vi "ColorImageTest.vi"() -> ()   [LabVIEW 2011]
uses:
  Microsoft.Kinect
  <vilib>/vision/NI_Vision_Development_Module.lvlib
panel:
  in  "ElevationAngle":i32 min=-27 max=27
  out "Iteration":i32
  in  "stop":bool
  in  "millisecondsWait":i32=1000
  out "error out":errorcluster
  out "Array":T1(array[cluster])
  out "Depth Frame":T2(plugin-control)
  out "BeamAngle":dbl
  out "SoundSourceAngle":dbl
  out "SoundSourceAngleConfidence":dbl
  out "Color Frame":T2(plugin-control)
  out "Color Pixel Data":u8[](array[numeric])
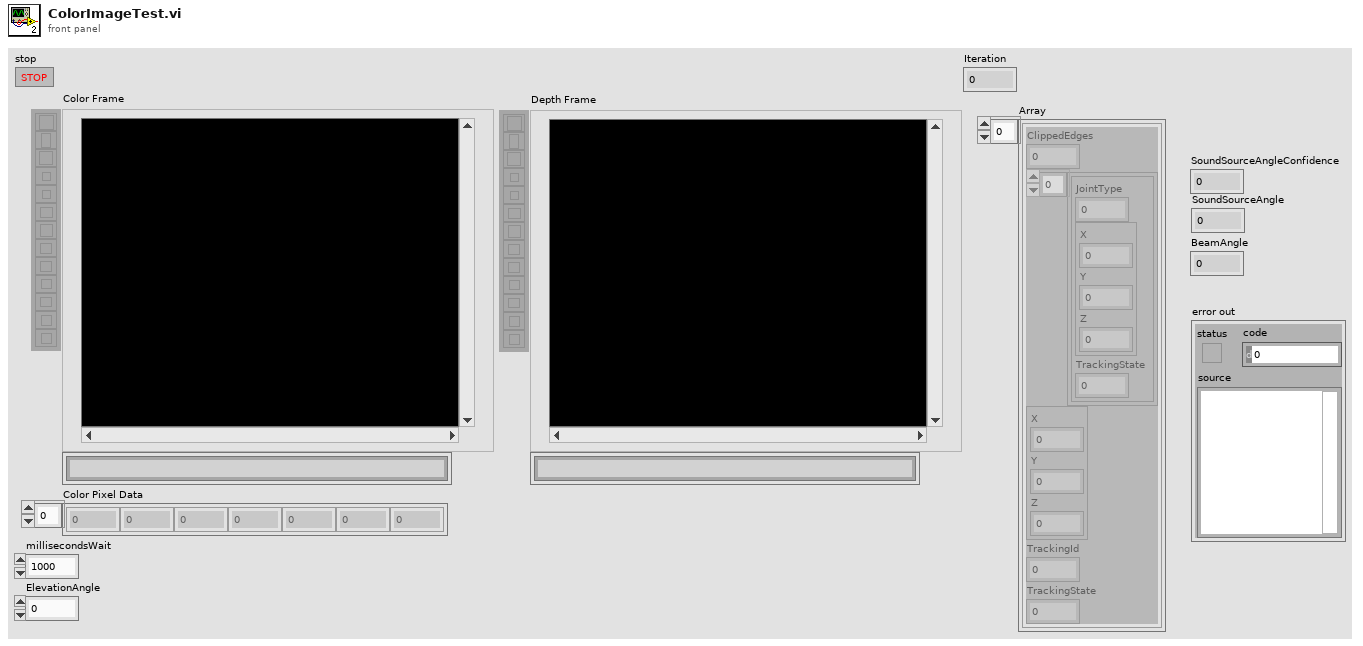
[diagram p1: front panel]
types:
  T1 = cluster{"ClippedEdges":i32, cluster{"JointType":i32, cluster{"X":sgl, "Y":sgl, "Z":sgl}, "TrackingState":i32}[], cluster{"X":sgl, "Y":sgl, "Z":sgl}, "TrackingId":i32, "TrackingState":i32}[]
  T2 = typedef "IMAQ Image.ctl" = refnum<image>
  T3 = typedef "Image Type" = u32
  T4 = cluster{"JointType":i32, cluster{"X":sgl, "Y":sgl, "Z":sgl}, "TrackingState":i32}
  T5 = cluster{"ClippedEdges":i32, cluster{"JointType":i32, cluster{"X":sgl, "Y":sgl, "Z":sgl}, "TrackingState":i32}[], cluster{"X":sgl, "Y":sgl, "Z":sgl}, "TrackingId":i32, "TrackingState":i32}
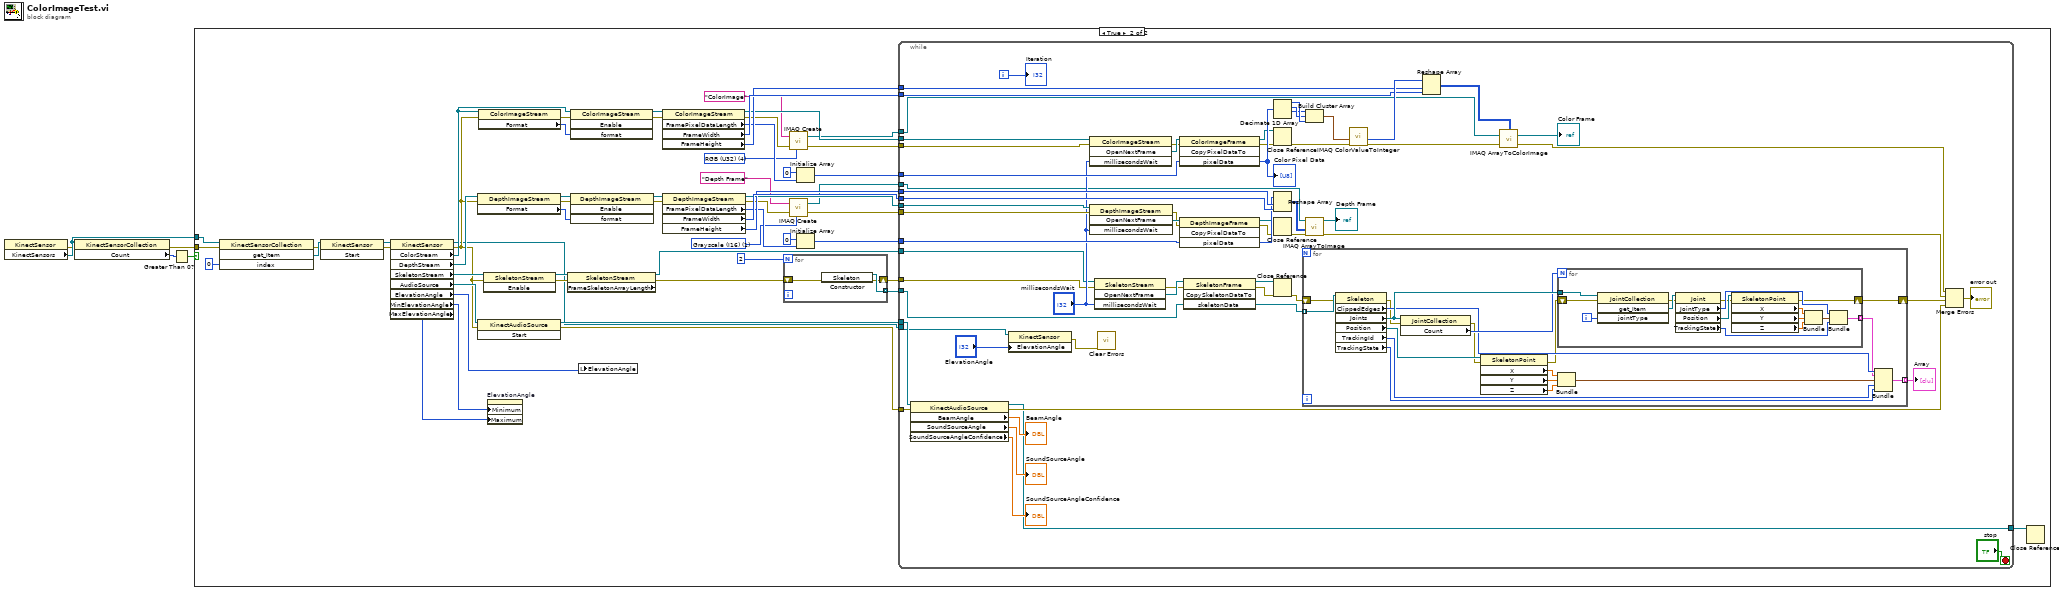
[diagram p0: block diagram]
diagram:
  n1 = property class="KinectSensor"() -> (error out=w2:errorcluster, "KinectSensors"=w5:refnum<k24>)  [unwired: 2 in, 1 out]
  n2 = property class="KinectSensorCollection"(reference=w5, error in=w2) -> (error out=w1:errorcluster, "Count"=w4:i32)  [unwired: 1 out]
  n3 = Greater Than 0?(x=w4) -> (x > 0?=w3:bool)
  n4 = case shown="True" w3 {
    tunnel: w5 -> [_ w62]
    tunnel: w1 -> [_ w48]
    frame False {
    }
    frame True {
      w19 = T3 4 items=["Grayscale (U8)", "Grayscale (I16)", "Grayscale (SGL)", "Complex (CSG)", "RGB (U32)", "HSL (U32)", "RGB (U64)", "Grayscale (U16)"] ("Image Type")
      w21 = T3 1 items=["Grayscale (U8)", "Grayscale (I16)", "Grayscale (SGL)", "Complex (CSG)", "RGB (U32)", "HSL (U32)", "RGB (U64)", "Grayscale (U16)"] ("Image Type")
      n5 = invoke class="KinectSensorCollection" method="get_Item"(reference=w62, error in=w48, "index"=0) -> (error out=w56:errorcluster, "get_Item"=w58:refnum<k24>)  [unwired: 1 in, 2 out]
      n6 = invoke class="KinectSensor" method="Start"(reference=w58, error in=w56) -> (reference out=w57:refnum<k24>, error out=w55:errorcluster)  [unwired: 1 in, 1 out]
      n7 = property class="KinectSensor"(reference=w57, error in=w55) -> (reference out=w9:refnum<k24>, error out=w44:errorcluster, "ColorStream"=w60:refnum<k24>, "DepthStream"=w53:refnum<k24>, "SkeletonStream"=w49:refnum<k24>, "AudioSource"=w47:refnum<k24>, "ElevationAngle"=w8:i32, "MinElevationAngle"=w7:i32, "MaxElevationAngle"=w6:i32)
      n8 = property class="DepthImageStream"(reference=w53, error in=w44) -> (reference out=w52:refnum<k24>, error out=w45:errorcluster, "Format"=w51:i32)
      n9 = invoke class="KinectAudioSource" method="Start"(reference=w47, error in=w44) -> (reference out=w50:refnum<k24>, error out=w46:errorcluster)  [unwired: 1 in, 1 out]
      n10 = property class="ColorImageStream"(reference=w60, error in=w44) -> (error out=w54:errorcluster, "Format"=w59:i32)  [unwired: 1 out]
      n11 = invoke class="SkeletonStream" method="Enable"(reference=w49, error in=w44) -> (reference out=w12:refnum<k24>, error out=w11:errorcluster)  [unwired: 1 in, 1 out]
      n12 = property on="ElevationAngle" class="DigNum (strict)"("Minimum"=w7, "Maximum"=w6) -> ()  [unwired: 2 in, 2 out]
      n13 = property class="SkeletonStream" props=["FrameSkeletonArrayLength"](reference=w12, error in=w11) -> (reference out=w15:refnum<k24>, error out=w14:errorcluster)  [unwired: 1 out]
      n14 = invoke class="DepthImageStream" method="Enable"(reference=w52, error in=w45, "format"=w51) -> (reference out=w34:refnum<k24>, error out=w37:errorcluster)  [unwired: 1 in, 2 out]
      n15 = invoke class="ColorImageStream" method="Enable"(reference=w60, error in=w54, "format"=w59) -> (reference out=w42:refnum<k24>, error out=w36:errorcluster)  [unwired: 1 in, 2 out]
      n16 = local write "ElevationAngle"(w8) -> ()
      n17 = property class="DepthImageStream"(reference=w34, error in=w37) -> (reference out=w33:refnum<k24>, error out=w23:errorcluster, "FramePixelDataLength"=w31:i32, "FrameWidth"=w39:i32, "FrameHeight"=w38:i32)
      n18 = property class="ColorImageStream"(reference=w42, error in=w36) -> (reference out=w35:refnum<k24>, error out=w18:errorcluster, "FramePixelDataLength"=w28:i32, "FrameWidth"=w41:i32, "FrameHeight"=w40:i32)
      n19 = for {
        N: 2 -> [_]
        tunnel: [w159] -> w43 mode=indexing
        shift-right: [w157] -> w13
        shift-left: w14 -> [w158]
        n20 = constructor class="Skeleton"(error in=w158) -> (reference out=w159:refnum<k24>, error out=w157:errorcluster)  [unwired: 2 in, 1 out]
      }
      n21 = call "IMAQ Create"("Image Name"="ColorImage", "Image Type"=w19, "error in (no error)"=w18) -> ("New Image"=w16:T2, "error out"=w17:errorcluster)  [unwired: 2 in]
      n22 = call "IMAQ Create"("Image Name"="Depth Frame", "Image Type"=w21, "error in (no error)"=w23) -> ("New Image"=w24:T2, "error out"=w22:errorcluster)  [unwired: 2 in]
      n23 = Initialize Array(u8 0, w28) -> (w27:u8[])
      n24 = Initialize Array(i16 0, w31) -> (w30:i16[])
      n25 = while {
        tunnel: w15 -> [w66]
        tunnel: w50 -> [w123]
        tunnel: w46 -> [w122]
        tunnel: w13 -> [w67]
        tunnel: w43 -> [w121]
        tunnel: w41 -> [w102]
        tunnel: w40 -> [w101]
        tunnel: w39 -> [w99]
        tunnel: w38 -> [w98]
        tunnel: w22 -> [w97]
        tunnel: w35 -> [w96]
        tunnel: w17 -> [w95]
        tunnel: w33 -> [w94]
        tunnel: w30 -> [w89]
        tunnel: w27 -> [w91]
        tunnel: [w80] -> w26
        tunnel: w24 -> [w75]
        tunnel: w16 -> [w73]
        tunnel: w9 -> [w65]
        i -> [w92]
        stop <- "stop" stop-if-true
        n26 = property class="KinectAudioSource"(reference=w123, error in=w122) -> (reference out=w80:refnum<k24>, error out=w106:errorcluster, "BeamAngle"=→"BeamAngle":dbl, "SoundSourceAngle"=→"SoundSourceAngle":dbl, "SoundSourceAngleConfidence"=→"SoundSourceAngleConfidence":dbl)
        n27 = property class="KinectSensor"(reference=w65, "ElevationAngle"="ElevationAngle") -> (error out=w63:errorcluster)  [unwired: 1 in, 1 out]
        n28 = invoke class="DepthImageStream" method="OpenNextFrame"(reference=w94, error in=w97, "millisecondsWait"="millisecondsWait") -> (error out=w87:errorcluster, "OpenNextFrame"=w90:refnum<k24>)  [unwired: 1 in, 2 out]
        n29 = invoke class="ColorImageStream" method="OpenNextFrame"(reference=w96, error in=w95, "millisecondsWait"="millisecondsWait") -> (error out=w100:errorcluster, "OpenNextFrame"=w120:refnum<k24>)  [unwired: 1 in, 2 out]
        n30 = invoke class="SkeletonStream" method="OpenNextFrame"(reference=w66, error in=w67, "millisecondsWait"="millisecondsWait") -> (error out=w110:errorcluster, "OpenNextFrame"=w111:refnum<k24>)  [unwired: 1 in, 2 out]
        n31 = call <vilib>:"Clear Errors.vi"("error in (no error)"=w63) -> ()  [unwired: 6 in, 1 out]
        n32 = invoke class="DepthImageFrame" method="CopyPixelDataTo"(reference=w90, error in=w87, "pixelData"=w89) -> (reference out=w77:refnum<k24>, error out=w76:errorcluster, "pixelData"=w88:i16[])  [unwired: 1 in, 1 out]
        n33 = invoke class="ColorImageFrame" method="CopyPixelDataTo"(reference=w120, error in=w100, "pixelData"=w91) -> (reference out=w79:refnum<k24>, error out=w78:errorcluster, "pixelData"=w119:u8[])  [unwired: 1 in, 1 out]
        "Color Pixel Data" <- w119
        n34 = invoke class="SkeletonFrame" method="CopySkeletonDataTo"(reference=w111, error in=w110, "skeletonData"=w121) -> (reference out=w69:refnum<k24>, error out=w71:errorcluster, "skeletonData"=w109:refnum<k24>[])  [unwired: 1 in, 1 out]
        n35 = Decimate 1D Array(w119) -> (w84:u8[], w83:u8[], w82:u8[])  [unwired: 1 out]
        n36 = Close Reference(reference=w79, error in (no error)=w78) -> (error out=w68:errorcluster)
        n37 = Reshape Array(w88, w98, w99) -> (w86:i16[][])
        n38 = Close Reference(reference=w77, error in (no error)=w76) -> (error out=w74:errorcluster)
        n39 = Close Reference(reference=w69, error in (no error)=w71) -> (error out=w70:errorcluster)
        n40 = for {
          tunnel: w109 -> [w141] mode=indexing
          tunnel: [w129] -> w108 mode=indexing
          shift-right: [w124] -> w107
          shift-left: w70 -> [w125]
          n41 = property class="Skeleton"(reference=w141, error in=w125) -> (error out=w128:errorcluster, "ClippedEdges"=w134:i32, "Joints"=w139:refnum<k24>, "Position"=w140:refnum<k24>, "TrackingId"=w131:i32, "TrackingState"=w130:i32)  [unwired: 1 out]
          n42 = property class="JointCollection"(reference=w139, error in=w128) -> (error out=w127:errorcluster, "Count"=w138:i32)  [unwired: 1 out]
          n43 = property class="SkeletonPoint"(reference=w140, error in=w127) -> (error out=w126:errorcluster, "X"=w137:sgl, "Y"=w136:sgl, "Z"=w135:sgl)  [unwired: 1 out]
          n44 = for {
            N: w138 -> [_]
            tunnel: w139 -> [w156]
            tunnel: [w146] -> w133 mode=indexing
            shift-right: [w142] -> w124
            shift-left: w126 -> [w145]
            i -> [w155]
            n45 = invoke class="JointCollection" method="get_Item"(reference=w156, error in=w145, "jointType"=w155) -> (error out=w144:errorcluster, "get_Item"=w154:refnum<k24>)  [unwired: 1 in, 2 out]
            n46 = property class="Joint"(reference=w154, error in=w144) -> (error out=w143:errorcluster, "JointType"=w149:i32, "Position"=w153:refnum<k24>, "TrackingState"=w147:i32)  [unwired: 1 out]
            n47 = property class="SkeletonPoint"(reference=w153, error in=w143) -> (error out=w142:errorcluster, "X"=w152:sgl, "Y"=w151:sgl, "Z"=w150:sgl)  [unwired: 1 out]
            n48 = Bundle("X"=w152, "Y"=w151, "Z"=w150) -> (w148:cluster{"X":sgl, "Y":sgl, "Z":sgl})  [unwired: 1 in]
            n49 = Bundle("JointType"=w149, w148, "TrackingState"=w147) -> (w146:T4)  [unwired: 1 in]
          }
          n50 = Bundle("X"=w137, "Y"=w136, "Z"=w135) -> (w132:cluster{"X":sgl, "Y":sgl, "Z":sgl})  [unwired: 1 in]
          n51 = Bundle("ClippedEdges"=w134, w133, w132, "TrackingId"=w131, "TrackingState"=w130) -> (w129:T5)  [unwired: 1 in]
        }
        "Array" <- w108
        n52 = Build Cluster Array(w82, w83, w84) -> (w81:cluster{u8, u8, u8}[])
        n53 = call "IMAQ ArrayToImage"("error in (no error)"=w74, "Image Pixels (I16)"=w86, "Image"=w75) -> ("error out"=w103:errorcluster, "Image Out"=→"Depth Frame":T2)  [unwired: 7 in]
        n54 = call "IMAQ ColorValueToInteger"("error in (no error)"=w68, "1D Color value array"=w81) -> ("1D U32 array"=w118:u32[], "error out"=w72:errorcluster)  [unwired: 3 in, 2 out]
        n55 = Reshape Array(w118, w101, w102) -> (w117:u32[][])
        n56 = call "IMAQ ArrayToColorImage"("Image Pixels (U32)"=w117, "Image"=w73, "error in (no error)"=w72) -> ("Image Out"=→"Color Frame":T2, "error out"=w112:errorcluster)  [unwired: 2 in]
        n57 = Merge Errors(w112, w103, w107, w106) -> (→"error out":errorcluster)
        "Iteration" <- w92
      }
      n58 = Close Reference(reference=w26) -> ()  [unwired: 1 in, 1 out]
    }
  }
